vi "手动调试界面.vi"() -> ()   [LabVIEW 2016, in "质控单元.lvlib"]
uses:
  <vilib>/Utility/miscctls.llb/LVPointTypeDef.ctl
panel:
  in  "CODCr柱塞泵加标":bool
  in  "CODMn柱塞泵加标":bool
  in  "氨氮柱塞泵加标":bool
  in  "总磷柱塞泵加标":bool
  in  "总氮柱塞泵加标":bool
  in  "总氮加标回收启动":bool
  in  "总氮停止":bool
  in  "总氮排液":bool
  in  "总氮调试":bool
  in  "CODCr加标回收启动":bool
  in  "CODCr停止":bool
  in  "CODCr排液":bool
  in  "CODCr调试":bool
  in  "CODMn加标回收启动":bool
  in  "CODMn停止":bool
  in  "CODMn排液":bool
  in  "CODMn调试":bool
  in  "总磷加标回收启动":bool
  in  "总磷停止":bool
  in  "总磷排液":bool
  in  "总磷调试":bool
  in  "氨氮加标回收启动":bool
  in  "氨氮停止":bool
  in  "氨氮排液":bool
  in  "氨氮调试":bool
  in  "关闭":bool
  # "手动调试界面"
  # "氨氮模块"
  # "总磷模块"
  # "总氮模块"
  # "CODMn模块"
  # "CODCr模块"
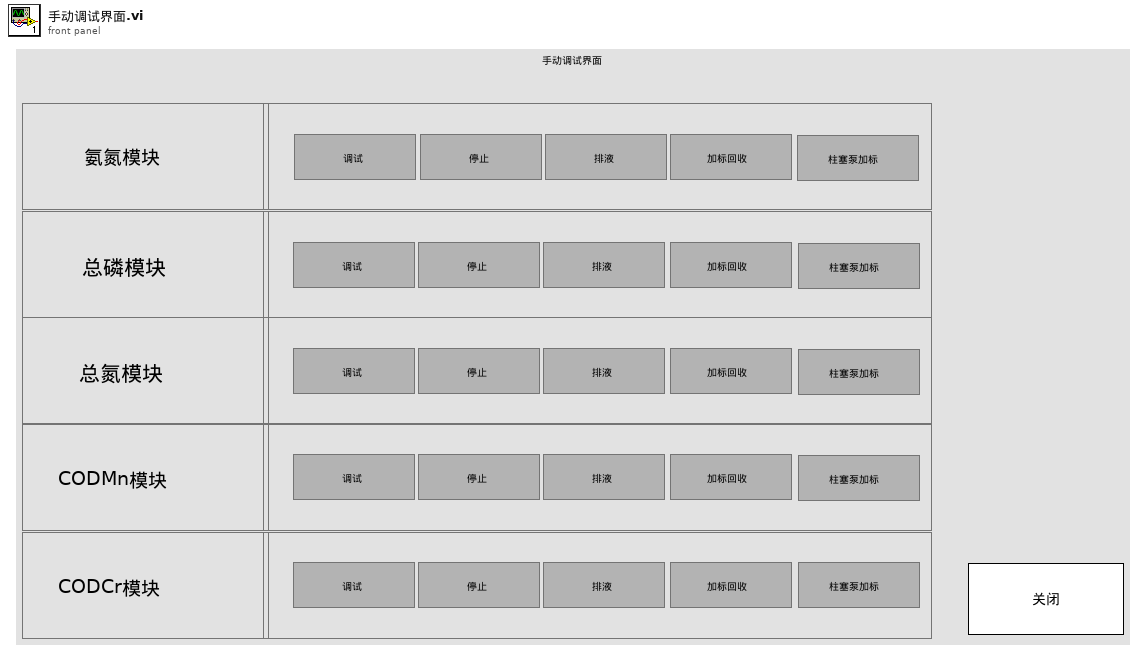
[diagram p1: front panel]
types:
  T1 = typedef "LVPointTypeDef.ctl" = cluster{"Horizontal":i16, "Vertical":i16}
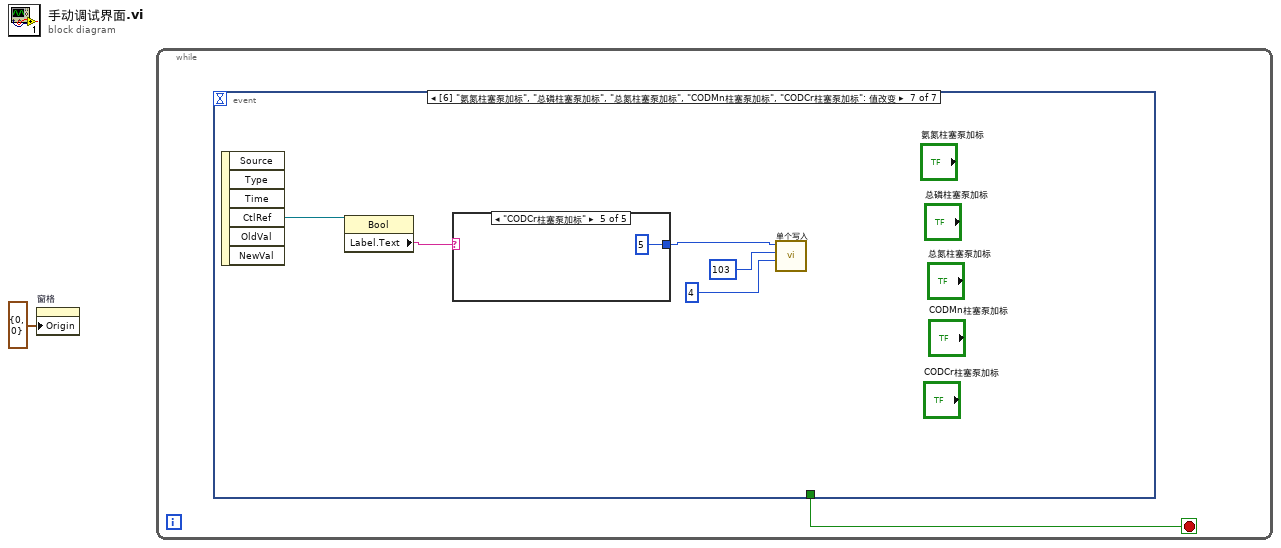
[diagram p0: block diagram]
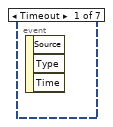
[diagram p2: hidden frame]
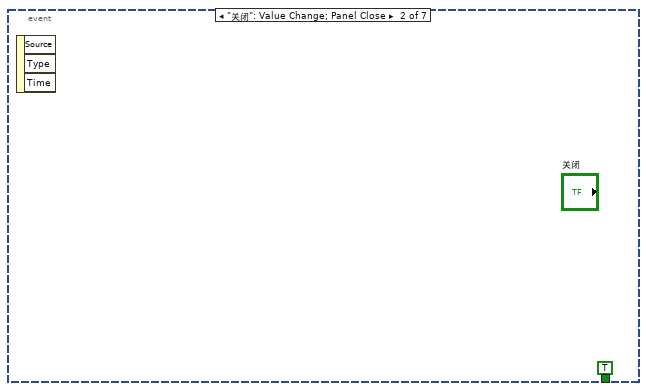
[diagram p3: hidden frame]
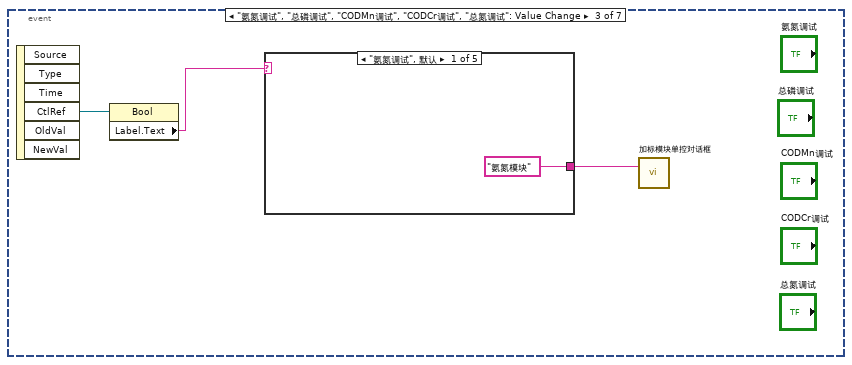
[diagram p4: hidden frame]
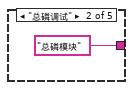
[diagram p5: hidden frame]
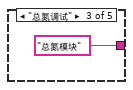
[diagram p6: hidden frame]
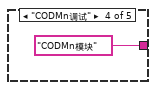
[diagram p7: hidden frame]
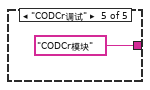
[diagram p8: hidden frame]
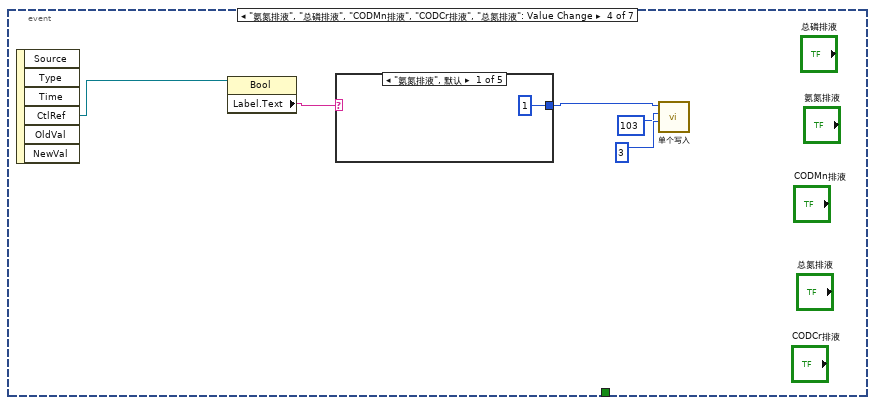
[diagram p9: hidden frame]
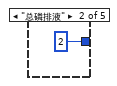
[diagram p10: hidden frame]
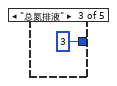
[diagram p11: hidden frame]
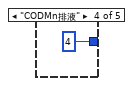
[diagram p12: hidden frame]
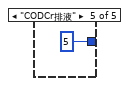
[diagram p13: hidden frame]
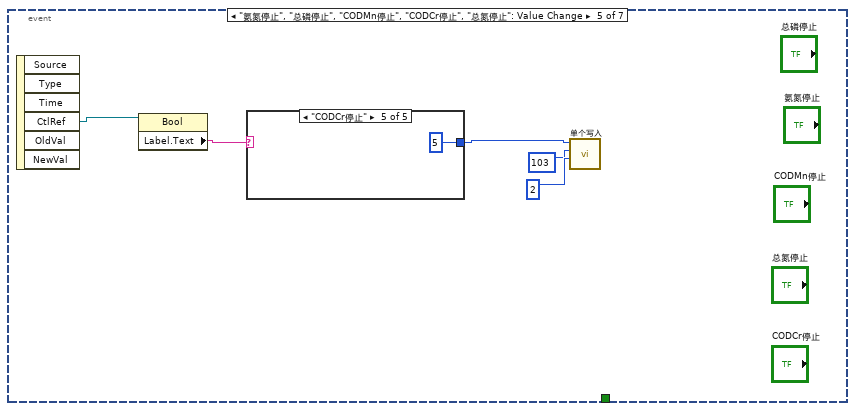
[diagram p14: hidden frame]
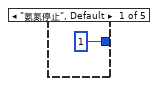
[diagram p15: hidden frame]
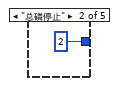
[diagram p16: hidden frame]
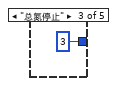
[diagram p17: hidden frame]
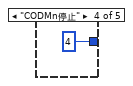
[diagram p18: hidden frame]
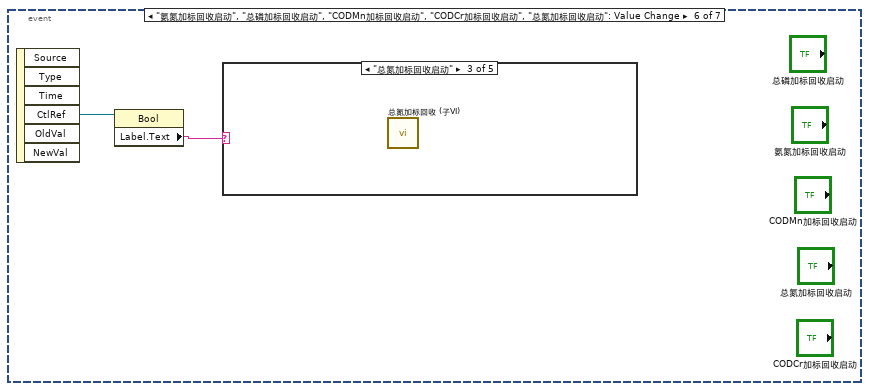
[diagram p19: hidden frame]
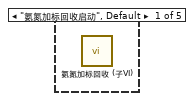
[diagram p20: hidden frame]
diagram:
  n1 = property on="窗格" class="Pane"("Origin"=T1 {"Horizontal"=0, "Vertical"=0} ("原点")) -> ()  [unwired: 2 in, 2 out]
  n2 = while {
    stop <- w2 stop-if-true
    n3 = event shown="[6] \"氨氮柱塞泵加标\", \"总磷柱塞泵加标\", \"总氮柱塞泵加标\", \"CODMn柱塞泵加标\", \"CODCr柱塞泵加标\": 值改变" {
      selector: _ -> [_ _ _ _ _ _ _]
      dyn-events: _ -> [_ _ _ _ _ _ _]
      timeout: _ -> [_ _ _ _ _ _ _]
      tunnel: [_ TRUE ("关闭") _ _ _ _ _] -> w2
      event Timeout {
        n4 = event-data() -> ()  [unwired: 1 in, 3 out]
      }
      event "关闭": Value Change; Panel Close {
        n5 = event-data() -> ()  [unwired: 1 in, 3 out]
      }
      event "氨氮调试", "总磷调试", "CODMn调试", "CODCr调试", "总氮调试": Value Change {
        n6 = event-data() -> ("CtlRef"=w5:refnum<vi>)  [unwired: 1 in, 5 out]
        n7 = property class="Bool"(reference=w5) -> ("Label.Text"=w4:string)  [unwired: 1 in, 2 out]
        n8 = case shown="\"氨氮调试\", 默认" w4 {
          tunnel: ["氨氮模块" ("标题") "总磷模块" ("标题") "总氮模块" ("标题") "CODMn模块" ("标题") "CODCr模块" ("标题")] -> w6
          frame "氨氮调试", Default {
          }
          frame "总磷调试" {
          }
          frame "总氮调试" {
          }
          frame "CODMn调试" {
          }
          frame "CODCr调试" {
          }
        }
        n9 = call "加标模块单控对话框.vi"("标题"=w6) -> ()  [unwired: 11 in]
      }
      event "氨氮排液", "总磷排液", "CODMn排液", "CODCr排液", "总氮排液": Value Change {
        n10 = event-data() -> ("CtlRef"=w12:refnum<vi>)  [unwired: 1 in, 5 out]
        n11 = property class="Bool"(reference=w12) -> ("Label.Text"=w16:string)  [unwired: 1 in, 2 out]
        n12 = case shown="\"氨氮排液\", 默认" w16 {
          tunnel: [u8 1 ("Slave ID") u8 2 ("Slave ID") u8 3 ("Slave ID") u8 4 ("Slave ID") u8 5 ("Slave ID")] -> w13
          frame "氨氮排液", Default {
          }
          frame "总磷排液" {
          }
          frame "总氮排液" {
          }
          frame "CODMn排液" {
          }
          frame "CODCr排液" {
          }
        }
        n13 = call "单个写入.vi"("value"=u16 3, "address"=u16 103, "Slave ID"=w13) -> ()  [unwired: 8 in, 1 out]
      }
      event "氨氮停止", "总磷停止", "CODMn停止", "CODCr停止", "总氮停止": Value Change {
        n14 = event-data() -> ("CtlRef"=w22:refnum<vi>)  [unwired: 1 in, 5 out]
        n15 = property class="Bool"(reference=w22) -> ("Label.Text"=w26:string)  [unwired: 1 in, 2 out]
        n16 = case shown="\"CODCr停止\"" w26 {
          tunnel: [u8 1 ("Slave ID") u8 2 ("Slave ID") u8 3 ("Slave ID") u8 4 ("Slave ID") u8 5 ("Slave ID")] -> w23
          frame "氨氮停止", Default {
          }
          frame "总磷停止" {
          }
          frame "总氮停止" {
          }
          frame "CODMn停止" {
          }
          frame "CODCr停止" {
          }
        }
        n17 = call "单个写入.vi"("value"=u16 2, "address"=u16 103, "Slave ID"=w23) -> ()  [unwired: 8 in, 1 out]
      }
      event "氨氮加标回收启动", "总磷加标回收启动", "CODMn加标回收启动", "CODCr加标回收启动", "总氮加标回收启动": Value Change {
        n18 = event-data() -> ("CtlRef"=w32:refnum<vi>)  [unwired: 1 in, 5 out]
        n19 = property class="Bool"(reference=w32) -> ("Label.Text"=w33:string)  [unwired: 1 in, 2 out]
        n20 = case shown="\"总氮加标回收启动\"" w33 {
          frame "氨氮加标回收启动", Default {
            n21 = call "氨氮加标回收 (子VI).vi"() -> ()  [unwired: 12 in]
          }
          frame "总磷加标回收启动" {
            n22 = call "总磷加标回收 (子VI).vi"() -> ()  [unwired: 12 in]
          }
          frame "总氮加标回收启动" {
            n23 = call "总氮加标回收 (子VI).vi"() -> ()  [unwired: 12 in]
          }
          frame "CODMn加标回收启动" {
            n24 = call "CODMn加标回收(子VI).vi"() -> ()  [unwired: 12 in]
          }
          frame "CODCr加标回收启动" {
            n25 = call "CODCr加标回收(子VI).vi"() -> ()  [unwired: 12 in]
          }
        }
      }
      event "氨氮柱塞泵加标", "总磷柱塞泵加标", "总氮柱塞泵加标", "CODMn柱塞泵加标", "CODCr柱塞泵加标": Value Change {
        n26 = event-data() -> ("CtlRef"=w34:refnum<vi>)  [unwired: 1 in, 5 out]
        n27 = property class="Bool"(reference=w34) -> ("Label.Text"=w38:string)  [unwired: 1 in, 2 out]
        n28 = case shown="\"CODCr柱塞泵加标\"" w38 {
          tunnel: [u8 1 ("Slave ID") u8 2 ("Slave ID") u8 3 ("Slave ID") u8 4 ("Slave ID") u8 5 ("Slave ID")] -> w35
          frame "氨氮柱塞泵加标", Default {
          }
          frame "总磷柱塞泵加标" {
          }
          frame "总氮柱塞泵加标" {
          }
          frame "CODMn柱塞泵加标" {
          }
          frame "CODCr柱塞泵加标" {
          }
        }
        n29 = call "单个写入.vi"("value"=u16 4, "address"=u16 103, "Slave ID"=w35) -> ()  [unwired: 8 in, 1 out]
      }
    }
  }
